vi "Process.vi"(8 "error in":errorcluster, 11 "Plugin in":refnum<class "MP750510.lvclass">) -> (0 "error out":errorcluster, 3 "Plugin out":refnum<class "MP750510.lvclass">)   [LabVIEW 2025, in "MP750510.lvlib" / "MP750510.lvclass"]
uses:
  MP750510.lvclass
  MP750510.lvclass/MP750510.ctl
  2d66c614-e823-4ffc-9934-4c28994fc39e.vi
  122693e4-a04a-460f-9438-fa59efd370a1.vi
  e2591670-10b9-4ebb-8b0e-9bd19a14f56b.vi
  4a5d90ae-e915-4044-ab01-9c82fceee7bf.vi
  f6c964ed-dc82-433e-8465-fbf78c16faac.vi
  <vilib>/FlexLogger/SDK/PluginSDK.lvlibp/PEFClasses/SDK/Channel/ParameterAccess/Read DBL.vi
  <vilib>/FlexLogger/SDK/PluginSDK.lvlibp/PEFClasses/SDK/Channel/ParameterAccess/Read Enum.vi
  <vilib>/FlexLogger/SDK/PluginSDK.lvlibp/PEFClasses/SDK/Channel/Channel.lvclass
  <vilib>/FlexLogger/SDK/PluginSDK.lvlibp/PEFClasses/SDK/Plugin/Plugin.lvclass
  3887ff43-7d63-4b53-9bff-e759e89904f9.vi
  3a89cda1-22df-451d-b168-bec7a3ec4817.vi
  71a2a187-dadd-4c60-ab06-7e6a51f94524.vi
  b3a5a46f-2055-4537-9b2b-eb3eadea12d4.vi
  7386d238-5a5d-4839-b5bc-669c0690fe74.vi
  C:/Program Files/National Instruments/LabVIEW 2025/vi.lib/FlexLogger/SDK/PluginSDK.lvlibp/PEFClasses/SDK/Plugin/Plugin.lvclass
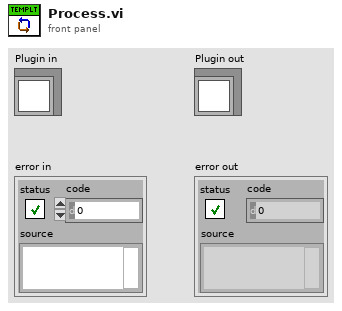
[diagram p1: front panel]
types:
  T1 = cluster{"Freq":dbl, "Amp":dbl, "Offset":dbl, "Phase":dbl, "Wave Type":enum16{"Sine", "Square", "Triangle", "Pulse", "Built In"}, "Initialised":bool}[]
  T2 = enum16{"Frequency", "Voltage Level", "Voltage Offset", "Phase", "Phase Sync", "Wave Type"}[]
  T3 = enum16{"Sine", "Square", "Triangle", "Pulse", "Built In"}
  T4 = enum16{"Frequency", "Voltage Level", "Voltage Offset", "Phase", "Phase Sync", "Wave Type"}
  T5 = cluster{"Freq":dbl, "Amp":dbl, "Offset":dbl, "Phase":dbl, "Wave Type":enum16{"Sine", "Square", "Triangle", "Pulse", "Built In"}, "Initialised":bool}
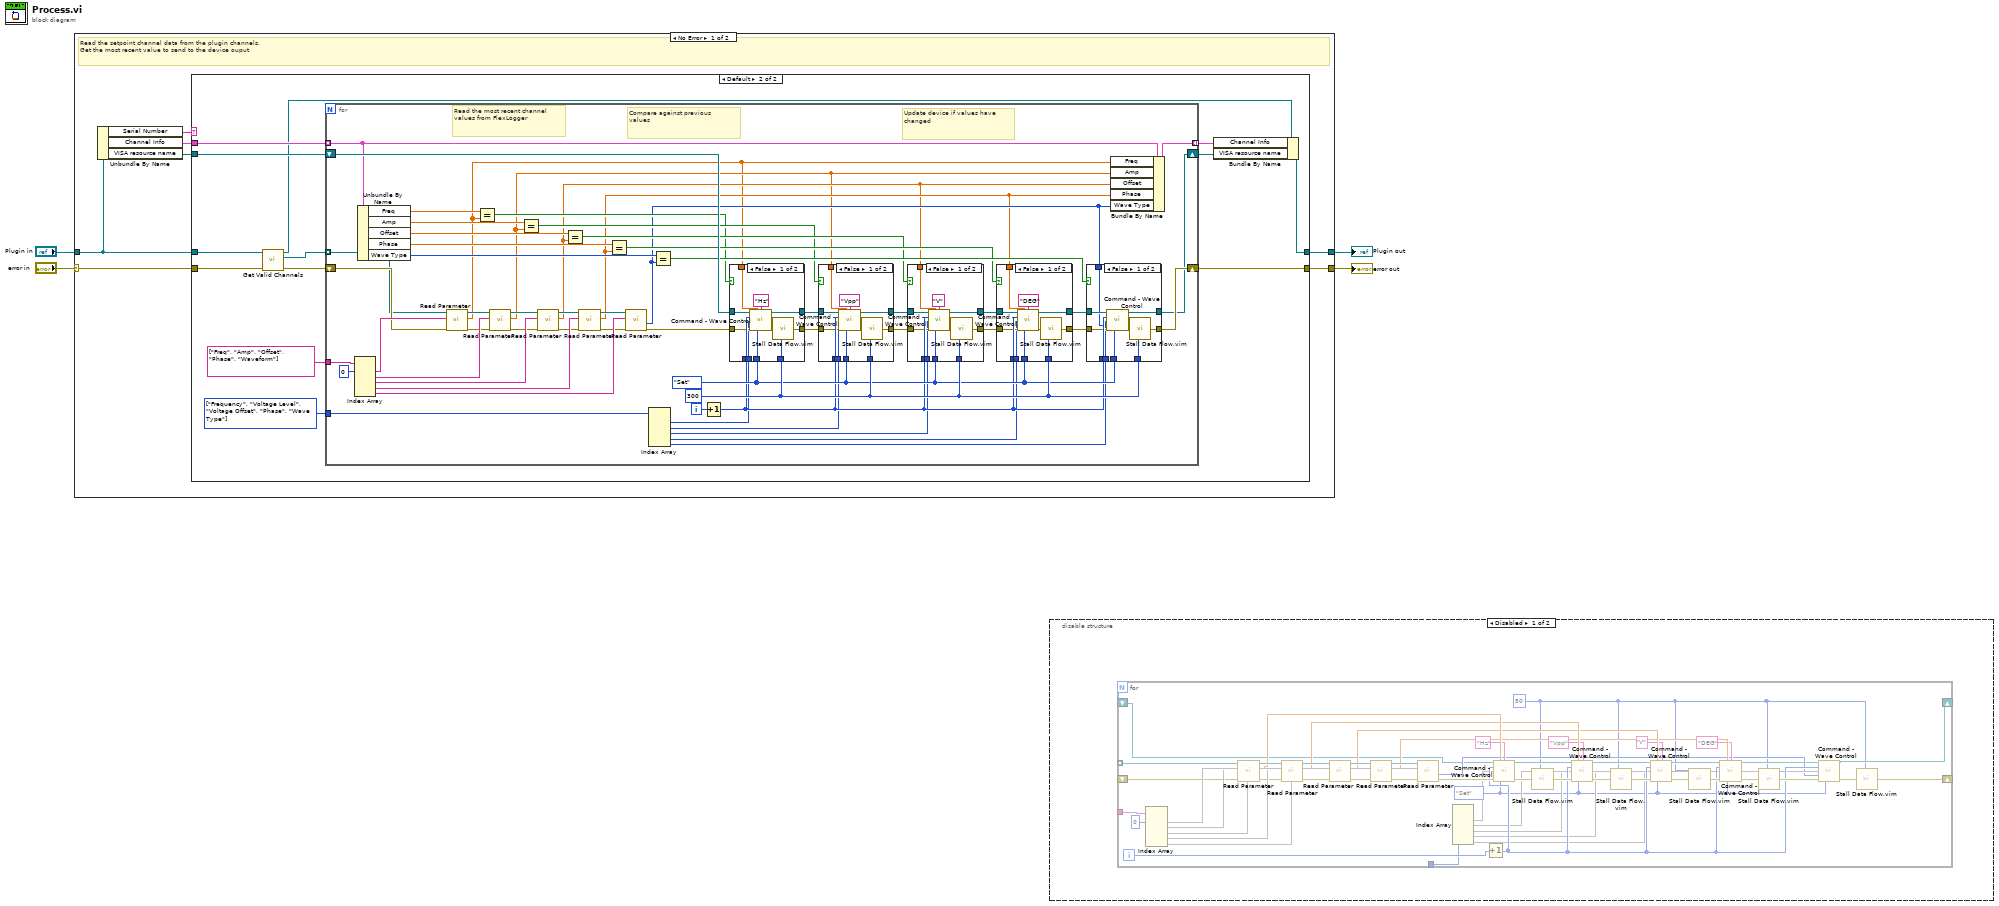
[diagram p0: block diagram]
diagram:
  n1 = case shown="No Error" "error in" {
    selector: "error in" -> [w9 w147]
    tunnel: [w5 w148] -> w4
    tunnel: "Plugin in" -> [w10 w148]
    tunnel: [w11 w147] -> w1
    frame No Error {
      # "Read the setpoint channel data from the plugin channels.\nGet the most recent value to send to the device ouput"
      n2 = Unbundle By Name(w10) -> ("Serial Number"=w8:string, "Channel Info"=w7:T1, "VISA resource name"=w6:refnum<visa-resource-name>)
      n3 = case shown="Default" w8 {
        tunnel: [w13 w26] -> w11
        tunnel: w10 -> [w12 w21]
        tunnel: w9 -> [w13 w20]
        tunnel: w7 -> [_ w19]
        tunnel: w6 -> [_ w18]
        tunnel: [w12 w14] -> w5
        frame "-" {
        }
        frame Default {
          w22 = T2 [enum."Frequency", enum."Voltage Level", enum."Voltage Offset", enum."Phase", enum."Wave Type"] items=["Frequency", "Voltage Level", "Voltage Offset", "Phase", "Phase Sync", "Wave Type"]
          n4 = call <vilib>:"Get Valid Channels.vi"("error in (no error)"=w20, "Plugin in"=w21) -> ("error out"=w23:errorcluster, "Channels"=w25:refnum<class "Channel.lvclass">[], "Plugin out"=w17:refnum<class "MP750510.lvclass">)  [unwired: 7 in]
          n5 = for {
            tunnel: w25 -> [w70] mode=indexing
            tunnel: string[] ["Freq", "Amp", "Offset", "Phase", "Waveform"] -> [w76]
            shift-right: [w48] -> w26
            shift-left: w23 -> [w75]
            tunnel: w22 -> [w47]
            shift-right: [w39] -> w15
            shift-left: w18 -> [w40]
            tunnel: w19 -> [w33] mode=indexing
            tunnel: [w32] -> w16 mode=indexing
            i -> [w45]
            w60 = u32 300 ("milliseconds to wait")
            w59 = enum16{"Set", "Get"}."Set" ("Command Type")
            # "Update device if values have changed"
            # "Compare against previous values"
            # "Read the most recent channel values from FlexLogger"
            n6 = Index Array(array=w76, index #1=0 ("index")) -> (element #1=w81:string, element #2=w80:string, element #3=w79:string, element #4=w78:string, element #5=w77:string)  [unwired: 4 in]
            n7 = Unbundle By Name(w33) -> ("Freq"=w65:dbl, "Amp"=w64:dbl, "Offset"=w63:dbl, "Phase"=w62:dbl, "Wave Type"=w61:T3)
            n8 = call-poly <vilib>:"Read Parameter.vi"("error in (no error)"=w75, "Name"=w81, "Channel in"=w70) -> ("error out"=w74:errorcluster, "Value"=w27:dbl, "Channel out"=w69:refnum<class "Channel.lvclass">)  [unwired: 5 in, 1 out]
            n9 = Equal?(x=w65, y=w27) -> (x = y?=w34:bool)
            n10 = call-poly <vilib>:"Read Parameter.vi"("error in (no error)"=w74, "Name"=w80, "Channel in"=w69) -> ("error out"=w73:errorcluster, "Value"=w28:dbl, "Channel out"=w68:refnum<class "Channel.lvclass">)  [unwired: 5 in, 1 out]
            n11 = Equal?(x=w64, y=w28) -> (x = y?=w35:bool)
            n12 = call-poly <vilib>:"Read Parameter.vi"("error in (no error)"=w73, "Name"=w79, "Channel in"=w68) -> ("error out"=w72:errorcluster, "Value"=w29:dbl, "Channel out"=w67:refnum<class "Channel.lvclass">)  [unwired: 5 in, 1 out]
            n13 = Equal?(x=w63, y=w29) -> (x = y?=w36:bool)
            n14 = call-poly <vilib>:"Read Parameter.vi"("error in (no error)"=w72, "Name"=w78, "Channel in"=w67) -> ("error out"=w71:errorcluster, "Value"=w30:dbl, "Channel out"=w66:refnum<class "Channel.lvclass">)  [unwired: 5 in, 1 out]
            n15 = Equal?(x=w62, y=w30) -> (x = y?=w37:bool)
            n16 = call-poly <vilib>:"Read Parameter.vi"("error in (no error)"=w71, "Name"=w77, "Channel in"=w66) -> ("error out"=w49:errorcluster, "Index"=w31:i32)  [unwired: 4 in, 3 out]
            n17 = Index Array(array=w47) -> (element #1=w46:T4, element #2=w44:T4, element #3=w43:T4, element #4=w42:T4, element #5=w41:T4)  [unwired: 5 in]
            n18 = Equal?(x=w61, y=w31) -> (x = y?=w38:bool)
            n19 = Increment(x=w45) -> (x+1=w54:i32)
            n20 = case shown="False" w34 {
              tunnel: w60 -> [w144 _]
              tunnel: w59 -> [w143 _]
              tunnel: [w142 w146] -> w58
              tunnel: w54 -> [w140 _]
              tunnel: [w139 w145] -> w50
              tunnel: w49 -> [w137 w145]
              tunnel: w46 -> [w136 _]
              tunnel: w40 -> [w135 w146]
              tunnel: w27 -> [w134 _]
              frame False {
                n21 = call "Command - Wave Control.vi"("VISA Refnum in"=w135, "Value"=w134, "Unit"="Hz", "Channel"=w140, "Command"=w136, "Error In"=w137, "Command Type"=w143) -> ("VISA Refnum out"=w142:refnum<visa-resource-name>, "Error Out"=w138:errorcluster)  [unwired: 6 in, 1 out]
                n22 = call "Stall Data Flow.vim"("value in"=w138, "milliseconds to wait"=w144) -> ("value out"=w139:errorcluster)  [unwired: 1 out]
              }
              frame True {
              }
            }
            n23 = case shown="False" w35 {
              tunnel: w60 -> [w131 _]
              tunnel: w59 -> [w130 _]
              tunnel: w58 -> [w129 w133]
              tunnel: [w128 w133] -> w57
              tunnel: w54 -> [w126 _]
              tunnel: [w125 w132] -> w51
              tunnel: w50 -> [w124 w132]
              tunnel: w44 -> [w122 _]
              tunnel: w28 -> [w121 _]
              frame False {
                n24 = call "Command - Wave Control.vi"("VISA Refnum in"=w129, "Value"=w121, "Unit"="Vpp", "Channel"=w126, "Command"=w122, "Error In"=w124, "Command Type"=w130) -> ("VISA Refnum out"=w128:refnum<visa-resource-name>, "Error Out"=w123:errorcluster)  [unwired: 6 in, 1 out]
                n25 = call "Stall Data Flow.vim"("value in"=w123, "milliseconds to wait"=w131) -> ("value out"=w125:errorcluster)  [unwired: 1 out]
              }
              frame True {
              }
            }
            n26 = case shown="False" w36 {
              tunnel: w60 -> [w118 _]
              tunnel: w59 -> [w117 _]
              tunnel: w57 -> [w116 w120]
              tunnel: [w115 w120] -> w56
              tunnel: w54 -> [w113 _]
              tunnel: [w112 w119] -> w52
              tunnel: w51 -> [w111 w119]
              tunnel: w43 -> [w109 _]
              tunnel: w29 -> [w108 _]
              frame False {
                n27 = call "Command - Wave Control.vi"("VISA Refnum in"=w116, "Value"=w108, "Unit"="V", "Channel"=w113, "Command"=w109, "Error In"=w111, "Command Type"=w117) -> ("VISA Refnum out"=w115:refnum<visa-resource-name>, "Error Out"=w110:errorcluster)  [unwired: 6 in, 1 out]
                n28 = call "Stall Data Flow.vim"("value in"=w110, "milliseconds to wait"=w118) -> ("value out"=w112:errorcluster)  [unwired: 1 out]
              }
              frame True {
              }
            }
            n29 = case shown="False" w37 {
              tunnel: w60 -> [w105 _]
              tunnel: w59 -> [w104 _]
              tunnel: w56 -> [w103 w107]
              tunnel: [w102 w107] -> w55
              tunnel: w54 -> [w100 _]
              tunnel: [w99 w106] -> w53
              tunnel: w52 -> [w98 w106]
              tunnel: w42 -> [w96 _]
              tunnel: w30 -> [w95 _]
              frame False {
                n30 = call "Command - Wave Control.vi"("VISA Refnum in"=w103, "Value"=w95, "Unit"="DEG", "Channel"=w100, "Command"=w96, "Error In"=w98, "Command Type"=w104) -> ("VISA Refnum out"=w102:refnum<visa-resource-name>, "Error Out"=w97:errorcluster)  [unwired: 6 in, 1 out]
                n31 = call "Stall Data Flow.vim"("value in"=w97, "milliseconds to wait"=w105) -> ("value out"=w99:errorcluster)  [unwired: 1 out]
              }
              frame True {
              }
            }
            n32 = case shown="False" w38 {
              tunnel: w60 -> [w92 _]
              tunnel: w59 -> [w91 _]
              tunnel: w55 -> [w90 w94]
              tunnel: w54 -> [w89 _]
              tunnel: w53 -> [w88 w93]
              tunnel: [w86 w93] -> w48
              tunnel: w41 -> [w85 _]
              tunnel: [w84 w94] -> w39
              tunnel: w31 -> [w83 _]
              frame False {
                n33 = call "Command - Wave Control.vi"("VISA Refnum in"=w90, "Channel"=w89, "Command"=w85, "Wave Type"=w83, "Error In"=w88, "Command Type"=w91) -> ("VISA Refnum out"=w84:refnum<visa-resource-name>, "Error Out"=w87:errorcluster)  [unwired: 7 in, 1 out]
                n34 = call "Stall Data Flow.vim"("value in"=w87, "milliseconds to wait"=w92) -> ("value out"=w86:errorcluster)  [unwired: 1 out]
              }
              frame True {
              }
            }
            n35 = Bundle By Name(cluster=w33, "Freq"=w27, "Amp"=w28, "Offset"=w29, "Phase"=w30, "Wave Type"=w31) -> (w32:T5)
          }
          n36 = Bundle By Name(cluster=w17, "Channel Info"=w16, "VISA resource name"=w15) -> (w14:refnum<class "MP750510.lvclass">)
        }
      }
    }
    frame Error {
    }
  }
  "error out" <- w1
  "Plugin out" <- w4
  n37 = disable-structure shown="Disabled" {
    frame Disabled {
      n38 = for {
        tunnel: _ -> [w189] mode=indexing
        tunnel: _ -> [w195]
        shift-right: [w174] -> _
        shift-left: _ -> [w194]
        tunnel: _ -> [w167]
        shift-right: [w151] -> _
        shift-left: _ -> [w152]
        i -> [w169]
        w149 = u32 50 ("milliseconds to wait")
        w150 = enum16{"Set", "Get"}."Set" ("Command Type")
        n39 = Index Array(array=w195, index #1=0 ("index")) -> (element #1=w200, element #2=w199, element #3=w198, element #4=w197, element #5=w196)  [unwired: 4 in]
        n40 = call-poly <vilib>:"Read Parameter.vi"("error in (no error)"=w194, "Name"=w200, "Channel in"=w189) -> ("error out"=w193:errorcluster, "Value"=w173:dbl, "Channel out"=w188:refnum<class "Channel.lvclass">)  [unwired: 5 in, 1 out]
        n41 = call-poly <vilib>:"Read Parameter.vi"("error in (no error)"=w193, "Name"=w199, "Channel in"=w188) -> ("error out"=w192:errorcluster, "Value"=w172:dbl, "Channel out"=w187:refnum<class "Channel.lvclass">)  [unwired: 5 in, 1 out]
        n42 = call-poly <vilib>:"Read Parameter.vi"("error in (no error)"=w192, "Name"=w198, "Channel in"=w187) -> ("error out"=w191:errorcluster, "Value"=w171:dbl, "Channel out"=w186:refnum<class "Channel.lvclass">)  [unwired: 5 in, 1 out]
        n43 = call-poly <vilib>:"Read Parameter.vi"("error in (no error)"=w191, "Name"=w197, "Channel in"=w186) -> ("error out"=w190:errorcluster, "Value"=w170:dbl, "Channel out"=w185:refnum<class "Channel.lvclass">)  [unwired: 5 in, 1 out]
        n44 = call-poly <vilib>:"Read Parameter.vi"("error in (no error)"=w190, "Name"=w196, "Channel in"=w185) -> ("error out"=w184:errorcluster, "Index"=w157:i32)  [unwired: 4 in, 3 out]
        n45 = Index Array(array=w167) -> (element #1=w166, element #2=w165, element #3=w164, element #4=w163, element #5=w162)  [unwired: 5 in]
        n46 = Increment(x=w169) -> (x+1=w168:i32)
        n47 = call "Command - Wave Control.vi"("VISA Refnum in"=w152, "Value"=w173, "Unit"="Hz", "Channel"=w168, "Command"=w166, "Error In"=w184, "Command Type"=w150) -> ("VISA Refnum out"=w153:refnum<visa-resource-name>, "Error Out"=w183:errorcluster)  [unwired: 6 in, 1 out]
        n48 = call "Stall Data Flow.vim"("value in"=w183, "milliseconds to wait"=w149) -> ("value out"=w178:errorcluster)  [unwired: 1 out]
        n49 = call "Command - Wave Control.vi"("VISA Refnum in"=w153, "Value"=w172, "Unit"="Vpp", "Channel"=w168, "Command"=w165, "Error In"=w178, "Command Type"=w150) -> ("VISA Refnum out"=w154:refnum<visa-resource-name>, "Error Out"=w182:errorcluster)  [unwired: 6 in, 1 out]
        n50 = call "Stall Data Flow.vim"("value in"=w182, "milliseconds to wait"=w149) -> ("value out"=w177:errorcluster)  [unwired: 1 out]
        n51 = call "Command - Wave Control.vi"("VISA Refnum in"=w154, "Value"=w171, "Unit"="V", "Channel"=w168, "Command"=w164, "Error In"=w177, "Command Type"=w150) -> ("VISA Refnum out"=w155:refnum<visa-resource-name>, "Error Out"=w181:errorcluster)  [unwired: 6 in, 1 out]
        n52 = call "Stall Data Flow.vim"("value in"=w181, "milliseconds to wait"=w149) -> ("value out"=w176:errorcluster)  [unwired: 1 out]
        n53 = call "Command - Wave Control.vi"("VISA Refnum in"=w155, "Value"=w170, "Unit"="DEG", "Channel"=w168, "Command"=w163, "Error In"=w176, "Command Type"=w150) -> ("VISA Refnum out"=w156:refnum<visa-resource-name>, "Error Out"=w180:errorcluster)  [unwired: 6 in, 1 out]
        n54 = call "Stall Data Flow.vim"("value in"=w180, "milliseconds to wait"=w149) -> ("value out"=w175:errorcluster)  [unwired: 1 out]
        n55 = call "Command - Wave Control.vi"("VISA Refnum in"=w156, "Channel"=w168, "Command"=w162, "Wave Type"=w157, "Error In"=w175, "Command Type"=w150) -> ("VISA Refnum out"=w151:refnum<visa-resource-name>, "Error Out"=w179:errorcluster)  [unwired: 7 in, 1 out]
        n56 = call "Stall Data Flow.vim"("value in"=w179, "milliseconds to wait"=w149) -> ("value out"=w174:errorcluster)  [unwired: 1 out]
      }
    }
    frame Enabled {
    }
  }
